vi "get_spawn_position.vi"(4 "error in":errorcluster, 5 "Vehicle Start Position":i32 min=-1 max=2 step=1, 6 "Starting Points":T6, 7 "simx in":T1={"Config"={"Trajectory"={"Number of frames"=0, "Frame number"=0, "Trajectory"=""}, "Weather"={"id"=""}}, "Connections"={"Simulator Connection"=refnum, "server_ip"="127.0.0.1", "Port"=0, "Sensor connections"=[]}, "Map"={"lanes"={"x"=[], "y"=[], "z"=[]}, "StartPosition"={"start_points"={"locations"=[], "rotations"=[], "type"=[]}, "StartRotation"=[], "StartLocation"=[]}, "Draw Map Size"={"Width"=0, "Height"=0}, "DrawArea"={"min_Y"=0.0, "min_X"=0.0, "Scale X"=0.0, "Scale Y"=0.0}, "Map"=bytes[0], "Map Geojson"=""}}) -> (0 "error out":errorcluster, 3 "simx out":T1={"Config"={"Trajectory"={"Number of frames"=0, "Frame number"=0, "Trajectory"=""}, "Weather"={"id"=""}}, "Connections"={"Simulator Connection"=refnum, "server_ip"="127.0.0.1", "Port"=0, "Sensor connections"=[]}, "Map"={"lanes"={"x"=[], "y"=[], "z"=[]}, "StartPosition"={"start_points"={"locations"=[], "rotations"=[], "type"=[]}, "StartRotation"=[], "StartLocation"=[]}, "Draw Map Size"={"Width"=0, "Height"=0}, "DrawArea"={"min_Y"=0.0, "min_X"=0.0, "Scale X"=0.0, "Scale Y"=0.0}, "Map"=bytes[0], "Map Geojson"=""}})   [LabVIEW 2019]
doc: "Obtain the start position and rotation for the vehicle from the available Starting Points."
uses:
  controls/start_points.ctl
  controls/simx_connection.ctl
  controls/config.ctl
  controls/trajectory.ctl
  controls/weather.ctl
  controls/connections.ctl
  <vilib>/Utility/miscctls.llb/LVBoundsTypeDef.ctl
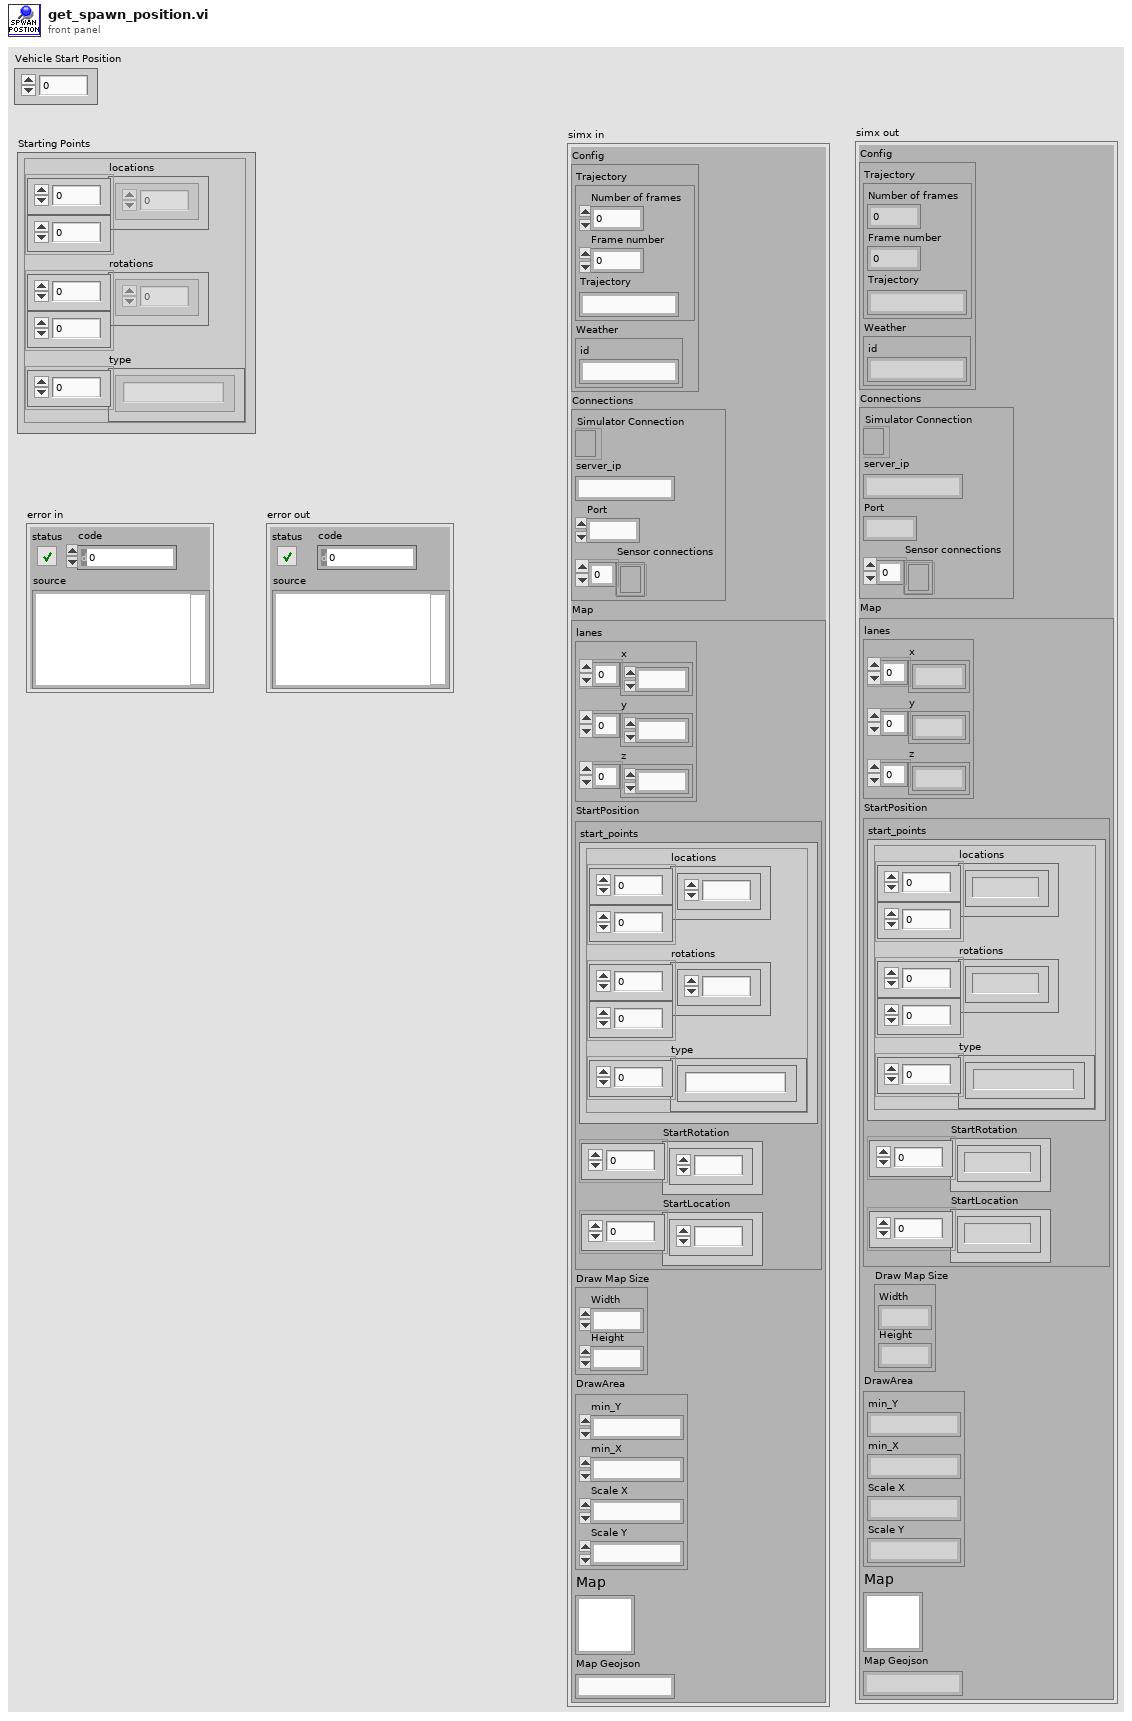
[diagram p1: front panel]
types:
  T1 = typedef "simx_connection.ctl" = cluster{"Config":T2, "Connections":T5, "Map":cluster{"lanes":cluster{"x":dbl[], "y":dbl[], "z":dbl[]}, "StartPosition":cluster{"start_points":T6, "StartRotation":dbl[], "StartLocation":dbl[]}, "Draw Map Size":T7, "DrawArea":cluster{"min_Y":dbl, "min_X":dbl, "Scale X":dbl, "Scale Y":dbl}, "Map":picture, "Map Geojson":string}}
  T2 = typedef "config.ctl" = cluster{"Trajectory":T3, "Weather":T4}
  T3 = typedef "trajectory.ctl" = cluster{"Number of frames":i32, "Frame number":i32, "Trajectory":string}
  T4 = typedef "weather.ctl" = cluster{"id":string}
  T5 = typedef "connections.ctl" = cluster{"Simulator Connection":refnum<k5>, "server_ip":string, "Port":i32, "Sensor connections":refnum<k5>[]}
  T6 = typedef "start_points.ctl" = cluster{"locations":dbl[][], "rotations":dbl[][], "type":string[]}
  T7 = typedef "LVBoundsTypeDef.ctl" = cluster{"Width":u32, "Height":u32}
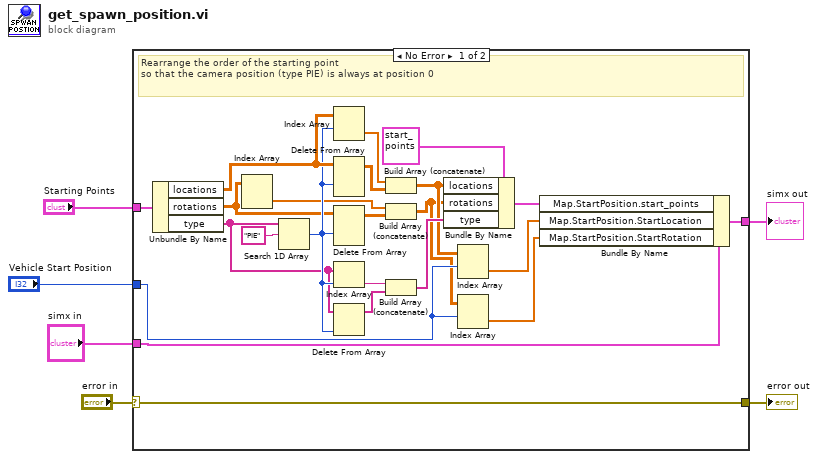
[diagram p0: block diagram]
diagram:
  n1 = case shown="No Error" "error in" {
    selector: "error in" -> [w12 w30]
    tunnel: "Starting Points" -> [w29 _]
    tunnel: [w14 w31] -> w1
    tunnel: "simx in" -> [w13 w31]
    tunnel: [w12 w30] -> w3
    tunnel: "Vehicle Start Position" -> [w10 _]
    frame No Error {
      # "Rearrange the order of the starting point \nso that the camera position (type PIE) is always at position 0"
      n2 = Unbundle By Name(w29) -> ("locations"=w28:dbl[][], "rotations"=w16:dbl[][], "type"=w22:string[])
      n3 = Index Array(array=w16) -> (element=w19:dbl[])  [unwired: 2 in]
      n4 = Search 1D Array(1D array=w22, element="PIE") -> (index of element=w23:i32)  [unwired: 1 in]
      n5 = Index Array(array=w28, index (row)=w23) -> (element=w17:dbl[])  [unwired: 1 in]
      n6 = Delete From Array(array=w28, index (row)=w23) -> (array with subset deleted=w18:dbl[][])  [unwired: 2 in, 1 out]
      n7 = Delete From Array(array=w16, index (row)=w23) -> (array with subset deleted=w20:dbl[][])  [unwired: 2 in, 1 out]
      n8 = Index Array(array=w22, index=w23) -> (element=w24:string)
      n9 = Delete From Array(array=w22, index=w23) -> (array with subset deleted=w25:string[])  [unwired: 1 in, 1 out]
      n10 = Build Array (concatenate)(w17, w18) -> (w8:dbl[][])
      n11 = Build Array (concatenate)(w19, w20) -> (w7:dbl[][])
      n12 = Build Array (concatenate)(w24, w25) -> (w26:string[])
      n13 = Bundle By Name(cluster=T6 {"locations"=[[5550.0, 310.0, 20.0], [12760.0, 2400.0, 20.0], [13490.0, 8590.0, 102.0], [22098.00390625, 3977.90283203125, 415.6770935058594]], "rotations"=[[0.0, 0.0, 0.0], [0.0, 0.0, 0.0], [0.0, 0.0, 0.0], [-0.4340515434741974, -14.976520538330078, 0.0]], "type"=["startPlayer", "startPlayer", "startPlayer", "PIE"]} ("start_points 2"), "locations"=w8, "rotations"=w7, "type"=w26) -> (w27:T6)
      n14 = Index Array(array=w8, index (row)=w10) -> (element=w11:dbl[])  [unwired: 1 in]
      n15 = Index Array(array=w7, index (row)=w10) -> (element=w9:dbl[])  [unwired: 1 in]
      n16 = Bundle By Name(cluster=w13, "Map.StartPosition.start_points"=w27, "Map.StartPosition.StartLocation"=w11, "Map.StartPosition.StartRotation"=w9) -> (w14:T1)
    }
    frame Error {
    }
  }
  "simx out" <- w1
  "error out" <- w3
